vi "Stop OPC UA.vi"(8 "error in (no error)":errorcluster, 11 "SM EOL Station Actor in":refnum<class "OPC Server.lvclass">) -> (0 "error out":errorcluster, 3 "SM EOL Station Actor out":refnum<class "OPC Server.lvclass">)   [LabVIEW 2021, in "OPC Server.lvlib" / "OPC Server.lvclass"]
uses:
  OPC Server.lvclass
  OPC Server.lvclass/OPC Server.ctl
  <vilib>/OPCUA/NI OPC UA Server.lvlib
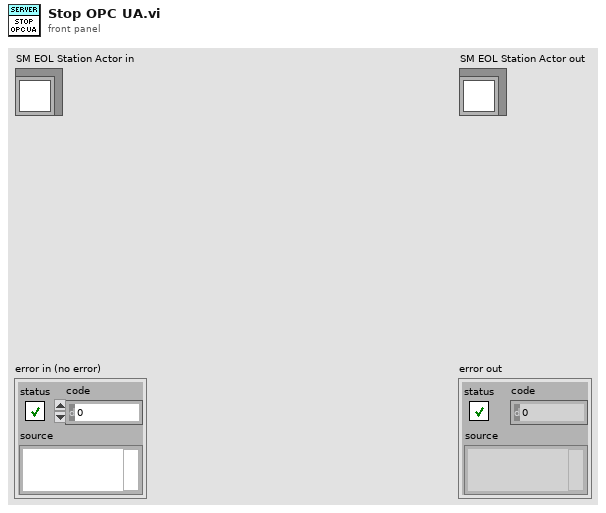
[diagram p1: front panel]
types:
  T1 = typedef "NodeId.ctl" = string
  T2 = typedef "OPC UA Server Refnum.ctl" = refnum<k21>
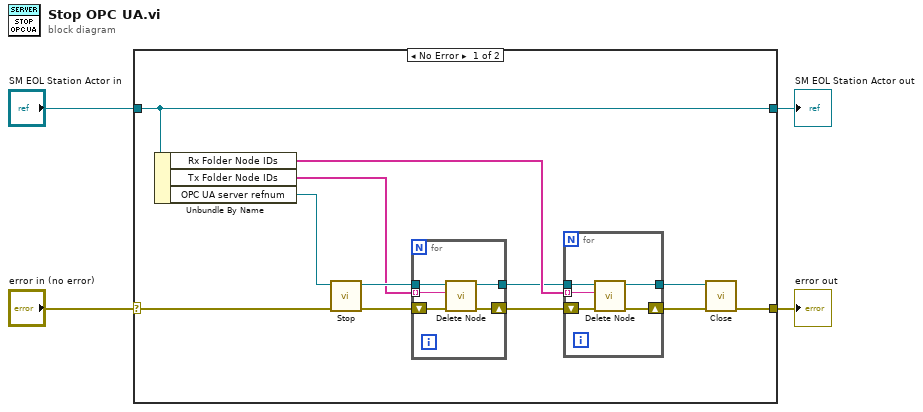
[diagram p0: block diagram]
diagram:
  n1 = case shown="No Error" "error in (no error)" {
    selector: "error in (no error)" -> [w16 w28]
    tunnel: [w6 w28] -> w3
    tunnel: [w15 w27] -> w1
    tunnel: "SM EOL Station Actor in" -> [w15 w27]
    frame No Error {
      n2 = Unbundle By Name(w15) -> ("Rx Folder Node IDs"=w9:T1[], "Tx Folder Node IDs"=w11:T1[], "OPC UA server refnum"=w14:T2)
      n3 = call <vilib>:"Stop.vi"("error in (no error)"=w16, "OPC UA server refnum in"=w14) -> ("error out"=w13:errorcluster, "OPC UA server refnum out"=w12:T2)  [unwired: 8 in]
      n4 = for {
        tunnel: w11 -> [w22] mode=indexing
        shift-right: [w24] -> w10
        shift-left: w13 -> [w26]
        tunnel: w12 -> [w25]
        tunnel: [w23] -> w8
        n5 = call <vilib>:"Delete Node.vi"("error in (no error)"=w26, "node ID"=w22, "OPC UA server refnum in"=w25) -> ("error out"=w24:errorcluster, "OPC UA server refnum out"=w23:T2)  [unwired: 7 in]
      }
      n6 = for {
        tunnel: w9 -> [w17] mode=indexing
        shift-right: [w19] -> w7
        shift-left: w10 -> [w21]
        tunnel: w8 -> [w20]
        tunnel: [w18] -> w5
        n7 = call <vilib>:"Delete Node.vi"("error in (no error)"=w21, "node ID"=w17, "OPC UA server refnum in"=w20) -> ("error out"=w19:errorcluster, "OPC UA server refnum out"=w18:T2)  [unwired: 7 in]
      }
      n8 = call <vilib>:"Close.vi"("error in (no error)"=w7, "OPC UA server refnum in"=w5) -> ("error out"=w6:errorcluster)  [unwired: 9 in]
    }
    frame Error {
    }
  }
  "error out" <- w3
  "SM EOL Station Actor out" <- w1
